vi "TestQR2.vi"() -> ()   [LabVIEW 2017]
uses:
  <vilib>/userdefined/High Color/IMAQdx.ctl
  <vilib>/vision/driver/NI_Vision_Acquisition_Software.lvlib
  <resource>/objmgr/imaqdx.rc
panel:
  out "standard output":string
  out "Image Out":T1(plugin-control)
  out "x-y":dbl
  in  "stop":bool
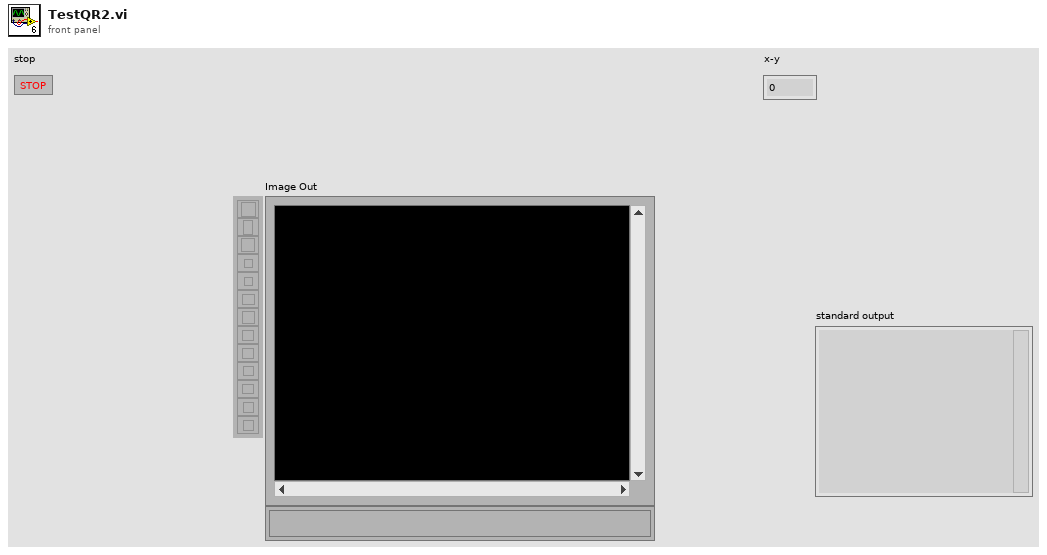
[diagram p1: front panel]
types:
  T1 = typedef "IMAQ Image.ctl" = refnum<image>
  T2 = typedef "IMAQdx.ctl" = refnum<k21>
  T3 = cluster{"Video Mode":u32, "Video Mode Name":string}[]
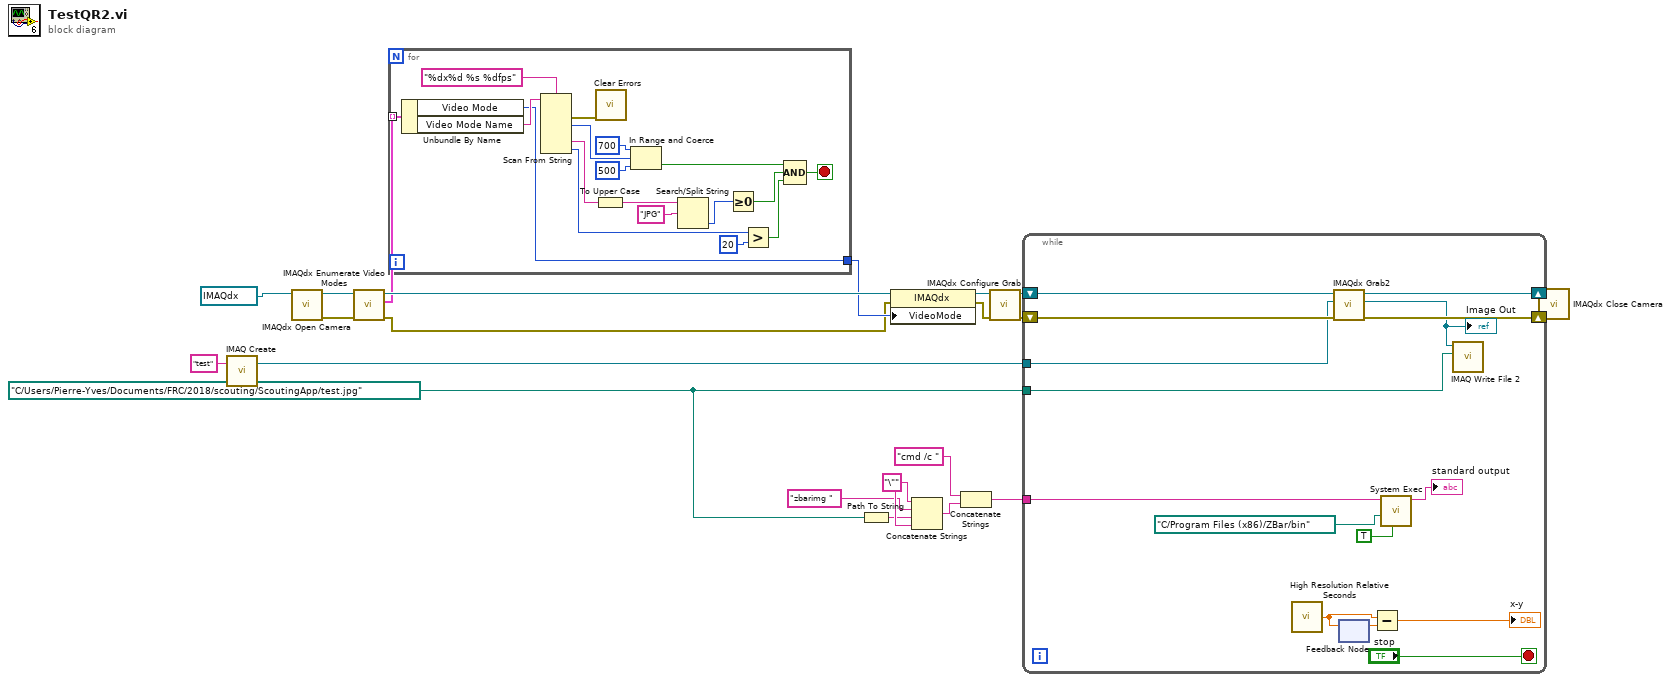
[diagram p0: block diagram]
diagram:
  w6 = path "C:/Users/Pierre-Yves/Documents/FRC/2018/scouting/ScoutingApp/test.jpg" ("File Path")
  w10 = "\"" ("string")
  n1 = call "IMAQ Create"("Image Name"="test") -> ("New Image"=w18:T1)  [unwired: 4 in, 1 out]
  n2 = call <vilib>:"IMAQdx Open Camera.vi"("Session In"=T2 "cam1") -> ("error out"=w13:errorcluster, "Session Out"=w15:T2)  [unwired: 9 in]
  n3 = call <vilib>:"IMAQdx Enumerate Video Modes.vi"("error in"=w13, "Session In"=w15) -> ("error out"=w2:errorcluster, "Video Modes"=w4:T3, "Session Out"=w14:T2)  [unwired: 6 in, 1 out]
  n4 = for {
    tunnel: w4 -> [w38] mode=indexing
    tunnel: [w24] -> w3
    stop <- w23 stop-if-true
    n5 = Unbundle By Name(w38) -> ("Video Mode"=w24:u32, "Video Mode Name"=w37:string)
    n6 = Scan From String(format string="%dx%d %s %dfps", input string=w37) -> (error out=w39:errorcluster, output 1=w30:i32, output 3=w36:string, output 4=w32:i32)  [unwired: 7 in, 2 out]
    n7 = To Upper Case(1:w36) -> (0:w34:string)
    n8 = call <vilib>:"Clear Errors.vi"("error in (no error)"=w39) -> ()  [unwired: 5 in, 2 out]
    n9 = In Range and Coerce(upper limit=700, x=w30, lower limit=500) -> (In Range?=w25:bool)  [unwired: 1 out]
    n10 = Search/Split String(string=w34, search string/char (-)="JPG") -> (offset of match=w33:i32)  [unwired: 1 in, 2 out]
    n11 = Greater Or Equal To 0?(x=w33) -> (x >= 0?=w26:bool)
    n12 = Greater?(x=w32, y=20) -> (0:w27:bool)
    n13 = Compound Arithmetic op=AND(w25, w26, w27) -> (w23:bool)
  }
  n14 = Path To String(path=w6) -> (string=w5:string)
  n15 = property class="IMAQdx"(reference=w14, error in=w2, "VideoMode"=w3) -> (reference out=w12:T2, error out=w1:errorcluster)
  n16 = Concatenate Strings(w10, "zbarimg " ("name or relative path"), w5, w10) -> (w11:string)
  n17 = Concatenate Strings("cmd /c " ("string"), w11) -> (w7:string)
  n18 = call <vilib>:"IMAQdx Configure Grab.vi"("error in"=w1, "Session In"=w12) -> ("error out"=w16:errorcluster, "Session Out"=w17:T2)  [unwired: 8 in]
  n19 = while {
    tunnel: w18 -> [w51]
    shift-right: [w52] -> w20
    shift-left: w17 -> [w55]
    shift-right: [w53] -> w21
    shift-left: w16 -> [w54]
    tunnel: w7 -> [w45]
    tunnel: w6 -> [w43]
    stop <- "stop" stop-if-true
    n20 = call <vilib>:"High Resolution Relative Seconds.vi"() -> ("relative seconds"=w48:dbl)
    n21 = call <vilib>:"IMAQdx Grab2.vi"("error in"=w54, "Image In"=w51, "Session In"=w55) -> ("error out"=w53:errorcluster, "Image Out"=w46:T1, "Session Out"=w52:T2)  [unwired: 5 in, 1 out]
    "Image Out" <- w46
    n22 = feedback #1() -> (w47:dbl)  [unwired: 1 in]
    n23 = feedback-in #1(w48) -> ()
    n24 = Subtract(x=w48, y=w47) -> (x-y=→"x-y":dbl)
    n25 = call <vilib>:"System Exec.vi"("run minimized? (F)"=TRUE, "working directory"=path "C:/Program Files (x86)/ZBar/bin", "command line"=w45) -> ("standard output"=→"standard output":string)  [unwired: 5 in, 3 out]
    n26 = call-poly "IMAQ Write File 2"("File Path"=w43, "Image"=w46) -> ()  [unwired: 8 in, 2 out]
  }
  n27 = call <vilib>:"IMAQdx Close Camera.vi"("error in"=w21, "Session In"=w20) -> ()  [unwired: 9 in, 1 out]
